vi "Register before Write.vi"(11 "Test Case In":refnum<class "Tests Event MessengerM.lvclass">) -> (0 "error out":errorcluster, 3 "Test Case Out":refnum<class "Tests Event MessengerM.lvclass">)   [LabVIEW 2020, in "Tests Event MessengerM.lvclass"]
uses:
  Tests Event MessengerM.lvclass
  <vilib>/Astemes/LUnit/Test Case.lvclass
  a782d602-5896-476d-8355-e9eda9a9c01b.vi
  2518f37c-463e-4735-b64c-b8e38770543d.vi
  993f4781-760c-4680-b53d-ed5056528a00.vi
  3c56c0a2-bcaa-4069-a73d-1b7303d1a380.vi
panel:
  out "msg 3":i32
  out "aborted? 3":bool
  out "aborted? 1":bool
  out "aborted? 0":bool
  out "msg 1":i32
  out "msg 0":i32
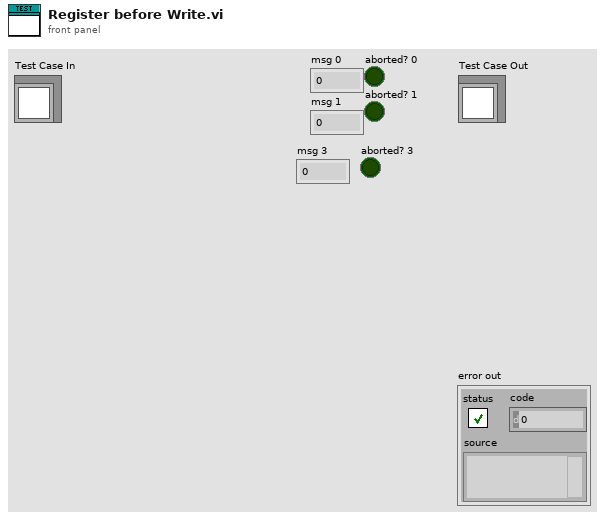
[diagram p1: front panel]
types:
  T1 = typedef "Event MessengerM-i32.lvlib/))Channel.ctl" = refnum<queue>
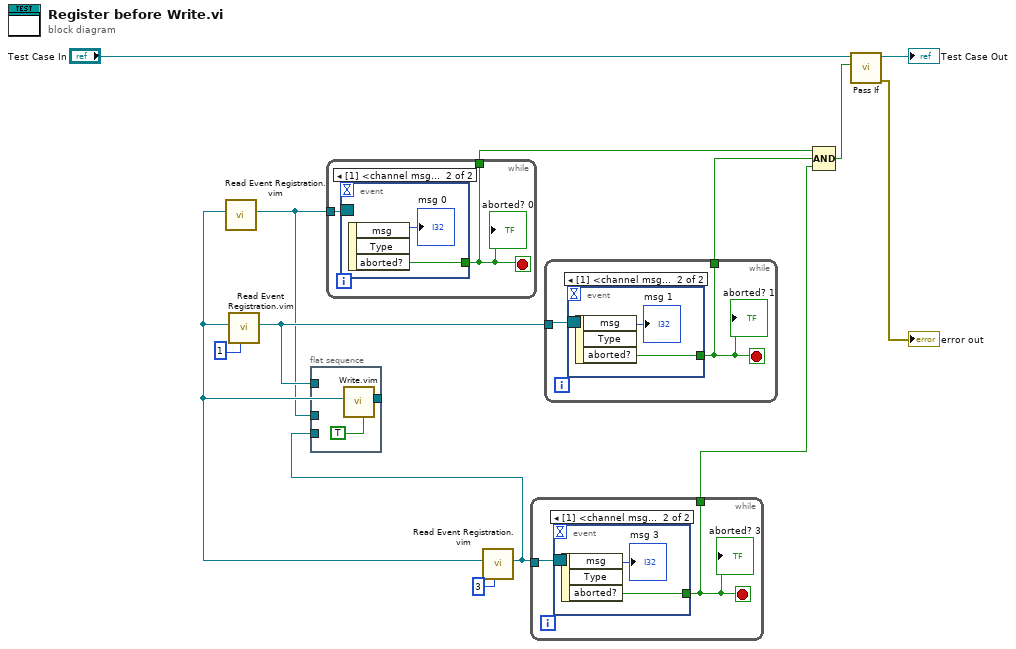
[diagram p0: block diagram]
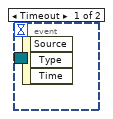
[diagram p2: hidden frame]
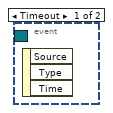
[diagram p3: hidden frame]
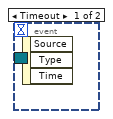
[diagram p4: hidden frame]
diagram:
  n1 = call "Read Event Registration.vim"("channel"=w6) -> ("event registration refnum"=w3:refnum<event-registration>)  [unwired: 10 in]
  n2 = call "Read Event Registration.vim"("subchannel"=1 ("subchannel (0)"), "channel"=w6) -> ("event registration refnum"=w10:refnum<event-registration>)  [unwired: 9 in]
  n3 = flat-sequence {
    tunnel: [w15] -> w6
    tunnel: w10 -> [_]
    tunnel: w4 -> [_]
    tunnel: w3 -> [_]
    frame #0 {
      n4 = call "Write.vim"("abort all (F)"=TRUE) -> ("channel"=w15:T1)  [unwired: 9 in, 1 out]
    }
  }
  n5 = while {
    tunnel: w3 -> [w17]
    tunnel: [w16] -> w7
    stop <- w16 stop-if-true
    n6 = event shown="[1] <channel msg>: User Event" {
      selector: w17 -> [_ _]
      dyn-events: _ -> [_ _]
      timeout: _ -> [_ _]
      tunnel: [_ w18] -> w16
      event Timeout {
        n7 = event-data() -> ()  [unwired: 1 in, 3 out]
      }
      event User Event {
        n8 = event-data() -> ("msg"=→"msg 0":i32, "aborted?"=w18:bool)  [unwired: 1 in, 1 out]
      }
    }
    "aborted? 0" <- w16
  }
  n9 = call "Read Event Registration.vim"("subchannel"=3 ("subchannel (0)"), "channel"=w6) -> ("event registration refnum"=w4:refnum<event-registration>)  [unwired: 9 in]
  n10 = while {
    tunnel: w4 -> [w21]
    tunnel: [w20] -> w5
    stop <- w20 stop-if-true
    n11 = event shown="[1] <channel msg>: User Event" {
      selector: w21 -> [_ _]
      dyn-events: _ -> [_ _]
      timeout: _ -> [_ _]
      tunnel: [_ w22] -> w20
      event Timeout {
        n12 = event-data() -> ()  [unwired: 1 in, 3 out]
      }
      event User Event {
        n13 = event-data() -> ("msg"=→"msg 3":i32, "aborted?"=w22:bool)  [unwired: 1 in, 1 out]
      }
    }
    "aborted? 3" <- w20
  }
  n14 = while {
    tunnel: w10 -> [w25]
    tunnel: [w24] -> w9
    stop <- w24 stop-if-true
    n15 = event shown="[1] <channel msg>: User Event" {
      selector: w25 -> [_ _]
      dyn-events: _ -> [_ _]
      timeout: _ -> [_ _]
      tunnel: [_ w26] -> w24
      event Timeout {
        n16 = event-data() -> ()  [unwired: 1 in, 3 out]
      }
      event User Event {
        n17 = event-data() -> ("msg"=→"msg 1":i32, "aborted?"=w26:bool)  [unwired: 1 in, 1 out]
      }
    }
    "aborted? 1" <- w24
  }
  n18 = Compound Arithmetic op=AND(w7, w9, w5) -> (w8:bool)
  n19 = call <vilib>:"Pass If.vi"("Pass?"=w8, "LUnit Test Case In"="Test Case In") -> ("error out"=→"error out":errorcluster, "LUnit Test Case Out"=→"Test Case Out":refnum<class "Tests Event MessengerM.lvclass">)  [unwired: 8 in]
